vi "image.vi"(7 "LabVIEW Web Service Request":refnum<class "Web Request.lvclass">) -> ()   [LabVIEW 2017]
uses:
  <vilib>/wsapi/Web Request.lvclass
  SystemController/SystemController.lvclass
panel:
  # "Use the Web Service Request input terminal to call the VIs on the Web Services palette. Do not remove it from the connector pane unless you don't need access to the palette."
  # "Each additional control wired to the connector pane will be available as an input in the URL. To include an indicator in terminal-mode output (the default setting), it must also be wired to the connector pane."
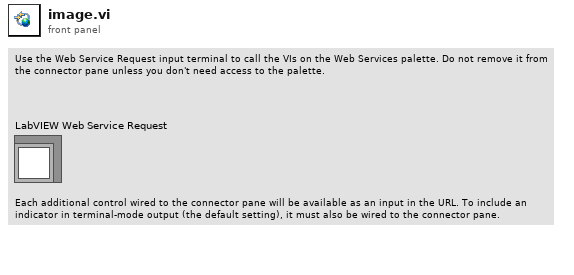
[diagram p1: front panel]
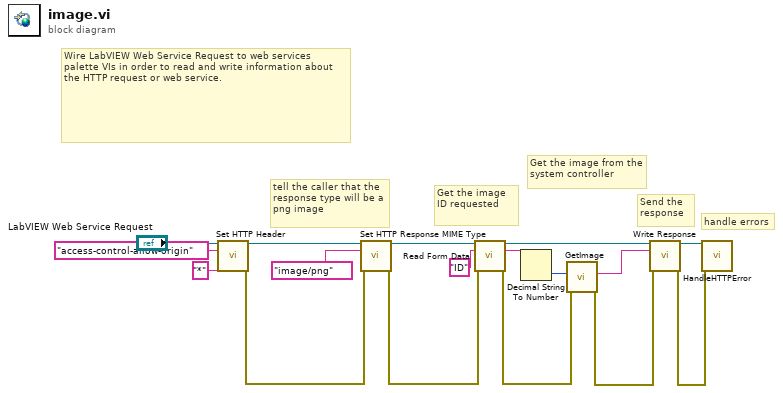
[diagram p0: block diagram]
diagram:
  # "Get the image ID requested"
  # "Send the response"
  # "Get the image from the system controller"
  # "tell the caller that the response type will be a png image"
  # "handle errors"
  # "Wire LabVIEW Web Service Request to web services palette VIs in order to read and write information about the HTTP request or web service."
  n1 = call <vilib>:"Set HTTP Header.vi"("LabVIEW Web Service Request"="LabVIEW Web Service Request", "header"="access-control-allow-origin", "header value"="*") -> ("LabVIEW Web Service Request out"=w4:refnum<class "Web Request.lvclass">, "error out"=w1:errorcluster)  [unwired: 11 in]
  n2 = call <vilib>:"Set HTTP Response MIME Type.vi"("LabVIEW Web Service Request"=w4, "MIME type (text/html)"="image/png", "error in (no error)"=w1) -> ("LabVIEW Web Service Request out"=w8:refnum<class "Web Request.lvclass">, "error out"=w7:errorcluster)  [unwired: 11 in]
  n3 = call <vilib>:"Read Form Data.vi"("LabVIEW Web Service Request"=w8, "key"="ID", "error in (no error)"=w7) -> ("LabVIEW Web Service Request out"=w10:refnum<class "Web Request.lvclass">, "value"=w12:string, "error out"=w6:errorcluster)  [unwired: 9 in, 1 out]
  n4 = Decimal String To Number(string=w12) -> (number=w11:i32)  [unwired: 2 in, 1 out]
  n5 = call "GetImage.vi"("error in (no error)"=w6, "index (0 = most recent)"=w11) -> ("error out"=w16:errorcluster, "Img"=w17:string)  [unwired: 8 in]
  n6 = call <vilib>:"Write Response.vi"("LabVIEW Web Service Request"=w10, "response string"=w17, "error in (no error)"=w16) -> ("LabVIEW Web Service Request out"=w15:refnum<class "Web Request.lvclass">, "error out"=w14:errorcluster)  [unwired: 11 in]
  n7 = call "HandleHTTPError.vi"("LabVIEW Web Service Request"=w15, "error in (no error)"=w14) -> ()  [unwired: 12 in, 2 out]
